vi "Write Parameters.vi"(8 "error in (no error)":errorcluster, 10 "Parameters":T1={"Skills"={"CirculateBall"={"rotationAngle"=86.0, "velocityFactor"=1.7, "OrientationFactor"=-1.0}, "ProtectBall"={"DistanceFromBall"=0.0}}, "TestSkill"=enum."CirculateBall"} {"Skills"."CirculateBall"."rotationAngle" format="%#_13g"}, 11 "Game in":refnum<class "Game.lvclass">) -> (0 "error out":errorcluster, 3 "Game out":refnum<class "Game.lvclass">)   [LabVIEW 2023, in "Game.lvclass"]
uses:
  Game.lvclass
  STP_Parameters/Parameters.ctl
  STP_Parameters/Skills.ctl
  Circulate_class/CIrculateSkillParameters.ctl
  STP_Parameters/TestSkills.ctl
  Game.lvclass/Game.ctl
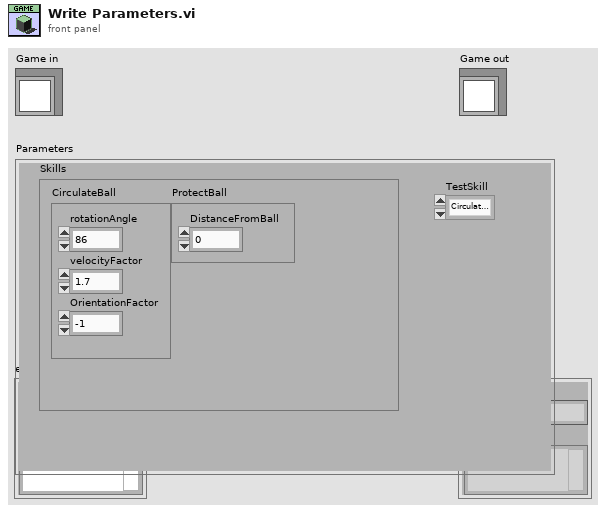
[diagram p1: front panel]
types:
  T1 = typedef "Parameters.ctl" = cluster{"Skills":T2, "TestSkill":T4}
  T2 = typedef "Skills.ctl" = cluster{"CirculateBall":T3, "ProtectBall":cluster{"DistanceFromBall":dbl}}
  T3 = typedef "CIrculateSkillParameters.ctl" = cluster{"rotationAngle":dbl, "velocityFactor":dbl, "OrientationFactor":dbl}
  T4 = typedef "TestSkills.ctl" = enum16{"CirculateBall", "ProtectBall", "ReceivePass", "GoTo"}
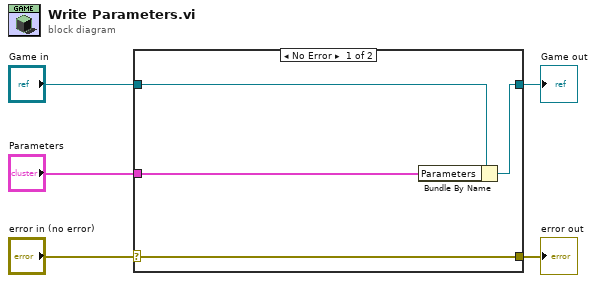
[diagram p0: block diagram]
diagram:
  n1 = case shown="No Error" "error in (no error)" {
    selector: "error in (no error)" -> [w9 w10]
    tunnel: [w9 w10] -> w4
    tunnel: [w7 w11] -> w2
    tunnel: "Game in" -> [w8 w11]
    tunnel: "Parameters" -> [w6 _]
    frame No Error {
      n2 = Bundle By Name(cluster=w8, "Parameters"=w6) -> (w7:refnum<class "Game.lvclass">)
    }
    frame Error {
    }
  }
  "error out" <- w4
  "Game out" <- w2
